vi "myRIOXGlobal.vi"() -> ()   [LabVIEW 2021]
uses:
  <vilib>/XNodeSupport/XNodeImage.ctl
  <vilib>/XNodeSupport/XNodeTerm4.ctl
  <vilib>/XNodeSupport/XNodeString.ctl
  <vilib>/XNodeSupport/XNodeVariant.ctl
  <vilib>/XNodeSupport/XNodeRect32.ctl
  <vilib>/XNodeSupport/XNodeInt.ctl
  <vilib>/XNodeSupport/XNodeBool.ctl
  <vilib>/XNodeSupport/XNodeTermDirection.ctl
  <vilib>/XNodeSupport/XNodeStandardHelpInfo.ctl
  <vilib>/XNodeSupport/XNodePath.ctl
  <vilib>/XNodeSupport/NI_XNodeSupport.lvlib
panel:
  out "AO Continuous Image":T1
  out "AO Continuous Help Info":T2={"Description"="Opens an FPGA reference to one or more analog output channels, which you use to perform continuous write operations. You must open a reference before you write values to an analog output channel.", "Path"=path "<helpdir>/elvis3vis.chm", "Tag"="elvis3vis_ao_continuous_sampling_open.html"}
  in  "AO Continuous Peripheral Name":string="AO (Continuous)"
  out "AI Continuous Image":T1
  out "AI Continuous Help Info":T2={"Description"="Opens an FPGA reference to one or more analog input channels, which you use to perform continuous read operations. You must open a reference before you read values from an analog input channel. ", "Path"=path "<helpdir>/elvis3vis.chm", "Tag"="myrioref_ai_continuous_sampling_open.html"}
  in  "AI Continuous Peripheral Name":string="AI (Continuous)"
  out "Max Range":T5={"Name"="Max Value", "Id"="Max Value", "Type"=variant(dbl[] []), "Bounds"={"Left"=16, "Top"=16, "Right"=24, "Bottom"=32}, "Input?"=TRUE, "Required?"=FALSE, "Recommended?"=TRUE, "Adaptive?"=FALSE, "Hidden?"=FALSE, "Direction"=enum."Auto", "Break Wire?"=FALSE, "English Name"=""}
  out "Min Range":T5={"Name"="Min Value", "Id"="Min Value", "Type"=variant(dbl[] []), "Bounds"={"Left"=8, "Top"=16, "Right"=16, "Bottom"=32}, "Input?"=TRUE, "Required?"=FALSE, "Recommended?"=TRUE, "Adaptive?"=FALSE, "Hidden?"=FALSE, "Direction"=enum."Auto", "Break Wire?"=FALSE, "English Name"=""}
  in  "Convert to SubVI OK Button":string="Convert"
  in  "Convert Fail Warning":string="Do you want to convert this VI to an empty VI? The current personality is incompatible with the peripheral. With an incompatible personality, you can only convert this VI to an empty VI."
  in  "Convert Success Warning":string="Do you want to convert this VI to a subVI? This operation disables error checking for FPGA personality at edit time."
  out "Timer IRQ Help Info":T2={"Description"="Creates timer interrupts.", "Path"=path "<helpdir>/myrioreference.chm", "Tag"="myrioref_create_timer_irq.html"}
  out "DI IRQ Help Info":T2={"Description"="Registers digital input interrupts.", "Path"=path "<helpdir>/myrioreference.chm", "Tag"="myrioref_register_di_irq.html"}
  out "AI IRQ Help Info":T2={"Description"="Registers analog input interrupts.", "Path"=path "<helpdir>/myrioreference.chm", "Tag"="myrioref_register_ai_irq.html"}
  in  "Timer IRQ Peripheral Name":string="Timer IRQ"
  in  "DI IRQ Peripheral Name":string="DI IRQ"
  in  "AI IRQ Peripheral Name":string="AI IRQ"
  out "Timer IRQ Image":T1
  out "DI IRQ Image":T1
  out "AI IRQ Image":T1
  out "DO Block Help Info":T2={"Description"="Opens a reference to one or more digital output channels, which you use to perform n samples write operations. You must open a reference before you write values to an digital output channel.", "Path"=path "<helpdir>/myrioreference.chm", "Tag"="myrioref_do_ns_open.html"}
  in  "DO Block Peripheral Name":string="DO (N Samples)"
  out "DO Block Image":T1
  out "DI Block Help Info":T2={"Description"="Opens a reference to one or more digital input channels, which you use to perform n samples write operations. You must open a reference before you read values from an digital input channel.", "Path"=path "<helpdir>/myrioreference.chm", "Tag"="myrioref_di_ns_open.html"}
  in  "DI Block Peripheral Name":string="DI (N Samples)"
  out "DI Block Image":T1
  out "AudioOut Block Help Info":T2={"Description"="Opens a reference to one or more audio output channels, which you use to perform n samples write operations. You must open a reference before you write values to an audio output channel.", "Path"=path "<helpdir>/myrioreference.chm", "Tag"="myrioref_audio_output_ns_open.html"}
  in  "AudioOut Block Peripheral Name":string="AudioOut (N Samples)"
  out "AudioOut Block Image":T1
  out "AudioIn Block Help Info":T2={"Description"="Opens a reference to one or more audio input channels, which you use to perform n samples read operations. You must open a reference before you read values from an audio input channel.", "Path"=path "<helpdir>/myrioreference.chm", "Tag"="myrioref_audio_input_ns_open.html"}
  in  "AudioIn Block Peripheral Name":string="AudioIn (N Samples)"
  out "AudioIn Block Image":T1
  out "AO Block Help Info":T2={"Description"="Opens a reference to one or more analog output channels, which you use to perform n samples write operations. You must open a reference before you write values to an analog output channel.", "Path"=path "<helpdir>/myrioreference.chm", "Tag"="myrioref_analog_output_ns_open.html"}
  in  "AO Block Peripheral Name":string="AO (N Samples)"
  out "AO Block Image":T1
  out "AI Block Help Info":T2={"Description"="Opens a reference to one or more analog input channels, which you use to perform n samples read operations. You must open a reference before you read values from an analog input channel.", "Path"=path "<helpdir>/myrioreference.chm", "Tag"="myrioref_analog_input_ns_open.html"}
  in  "AI Block Peripheral Name":string="AI (N Samples)"
  out "AI Block Image":T1
  out "SPI Help Info":T2={"Description"="Opens a reference to a serial peripheral interface (SPI) channel. You must open a reference before you use an SPI channel to write/read data to/from an SPI slave device.", "Path"=path "<helpdir>/myrioreference.chm", "Tag"="myrioref_spiopen.html"}
  out "PWM Help Info":T2={"Description"="Opens a reference to a pulse width modulation (PWM) channel. You must open a reference before you use a PWM channel to generate PWM signals.", "Path"=path "<helpdir>/myrioreference.chm", "Tag"="myrioref_pwmopen.html"}
  out "I2C Help Info":T2={"Description"="Opens a reference to an Inter-Integrated Circuit (I2C) channel. You must open a reference before you use an I2C channel to write/read data to/from an I2C slave device.", "Path"=path "<helpdir>/myrioreference.chm", "Tag"="myrioref_i2copen.html"}
  out "Encoder Help Info":T2={"Description"="Opens a reference to an encoder channel. You must open a reference before you use an encoder channel to read and decode signals from an encoder.", "Path"=path "<helpdir>/myrioreference.chm", "Tag"="myrioref_encoderopen.html"}
  out "DIO Help Info":T2={"Description"="Opens a reference to one or more digital I/O channels. You must open a reference before you read or write values.", "Path"=path "<helpdir>/myrioreference.chm", "Tag"="myrioref_dioopen.html"}
  out "AO Help Info":T2={"Description"="Opens a reference to one or more analog output channels. You must open a reference before you write values to an analog output channel.", "Path"=path "<helpdir>/myrioreference.chm", "Tag"="myrioref_aoopen.html"}
  out "AI Help Info":T2={"Description"="Opens a reference to one or more analog input channels. You must open a reference before you read values from an analog input channel.", "Path"=path "<helpdir>/myrioreference.chm", "Tag"="myrioref_aiopen.html"}
  out "Accelerometer Help Info":T2={"Description"="Opens a reference to one or more accelerometer channels. You must open a reference before you read values from an accelerometer channel.", "Path"=path "<helpdir>/myrioreference.chm", "Tag"="myrioref_accopen.html"}
  out "IP Address Term Constant":T5={"Name"="IP Address", "Id"="IP Address", "Type"=variant(string ""), "Bounds"={"Left"=0, "Top"=0, "Right"=8, "Bottom"=8}, "Input?"=TRUE, "Required?"=TRUE, "Recommended?"=FALSE, "Adaptive?"=FALSE, "Hidden?"=FALSE, "Direction"=enum."Auto", "Break Wire?"=FALSE, "English Name"=""}
  out "Allow Multiple Opens Term Constant":T5={"Name"="Allow multiple opens?", "Id"="Allow multiple opens?", "Type"=variant(bool FALSE), "Bounds"={"Left"=8, "Top"=0, "Right"=16, "Bottom"=16}, "Input?"=TRUE, "Required?"=FALSE, "Recommended?"=FALSE, "Adaptive?"=FALSE, "Hidden?"=FALSE, "Direction"=enum."Auto", "Break Wire?"=FALSE, "English Name"=""}
  out "Channel Names Term Constant":T5={"Name"="Channel Names", "Id"="Channel Names", "Type"=variant(tag[] []), "Bounds"={"Left"=0, "Top"=8, "Right"=8, "Bottom"=16}, "Input?"=TRUE, "Required?"=TRUE, "Recommended?"=FALSE, "Adaptive?"=FALSE, "Hidden?"=FALSE, "Direction"=enum."Auto", "Break Wire?"=FALSE, "English Name"=""}
  out "Channel Name Term Constant":T5={"Name"="Channel Name", "Id"="Channel Name", "Type"=variant(tag ""), "Bounds"={"Left"=0, "Top"=8, "Right"=8, "Bottom"=16}, "Input?"=TRUE, "Required?"=TRUE, "Recommended?"=FALSE, "Adaptive?"=FALSE, "Hidden?"=FALSE, "Direction"=enum."Auto", "Break Wire?"=FALSE, "English Name"=""}
  out "Error Out Term Constant":T5={"Name"="error out", "Id"="error out", "Type"=variant(errorcluster {"status"=FALSE, "code"=0, "source"=""}), "Bounds"={"Left"=24, "Top"=24, "Right"=32, "Bottom"=32}, "Input?"=FALSE, "Required?"=FALSE, "Recommended?"=TRUE, "Adaptive?"=FALSE, "Hidden?"=FALSE, "Direction"=enum."Auto", "Break Wire?"=FALSE, "English Name"=""}
  out "Error In Term Constant":T5={"Name"="error in (no error)", "Id"="error in (no error)", "Type"=variant(errorcluster {"status"=FALSE, "code"=0, "source"=""}), "Bounds"={"Left"=0, "Top"=24, "Right"=8, "Bottom"=32}, "Input?"=TRUE, "Required?"=FALSE, "Recommended?"=TRUE, "Adaptive?"=FALSE, "Hidden?"=FALSE, "Direction"=enum."Auto", "Break Wire?"=FALSE, "English Name"=""}
  in  "Error":string="The current personality or target does not support this VI."
  in  "Error Details":string="The current personality or target does not support this VI. Switch to another personality or change the current target."
  in  "SPI Peripheral Name":string="SPI"
  in  "PWM Peripheral Name":string="PWM"
  in  "I2C Peripheral Name":string="I2C"
  in  "Encoder Peripheral Name":string="Encoder"
  in  "AO Peripheral Name":string="AO"
  in  "DIO Peripheral Name":string="DIO"
  out "SPI Image":T1
  out "PWM Image":T1
  out "I2C Image":T1
  in  "Accelerometer Peripheral Name":string="Accelerometer"
  out "Accelerometer Image":T1
  in  "AI Peripheral Name":string="AI"
  out "Encoder Image":T1
  out "DIO Image":T1
  out "AO Image":T1
  out "AI Image":T1
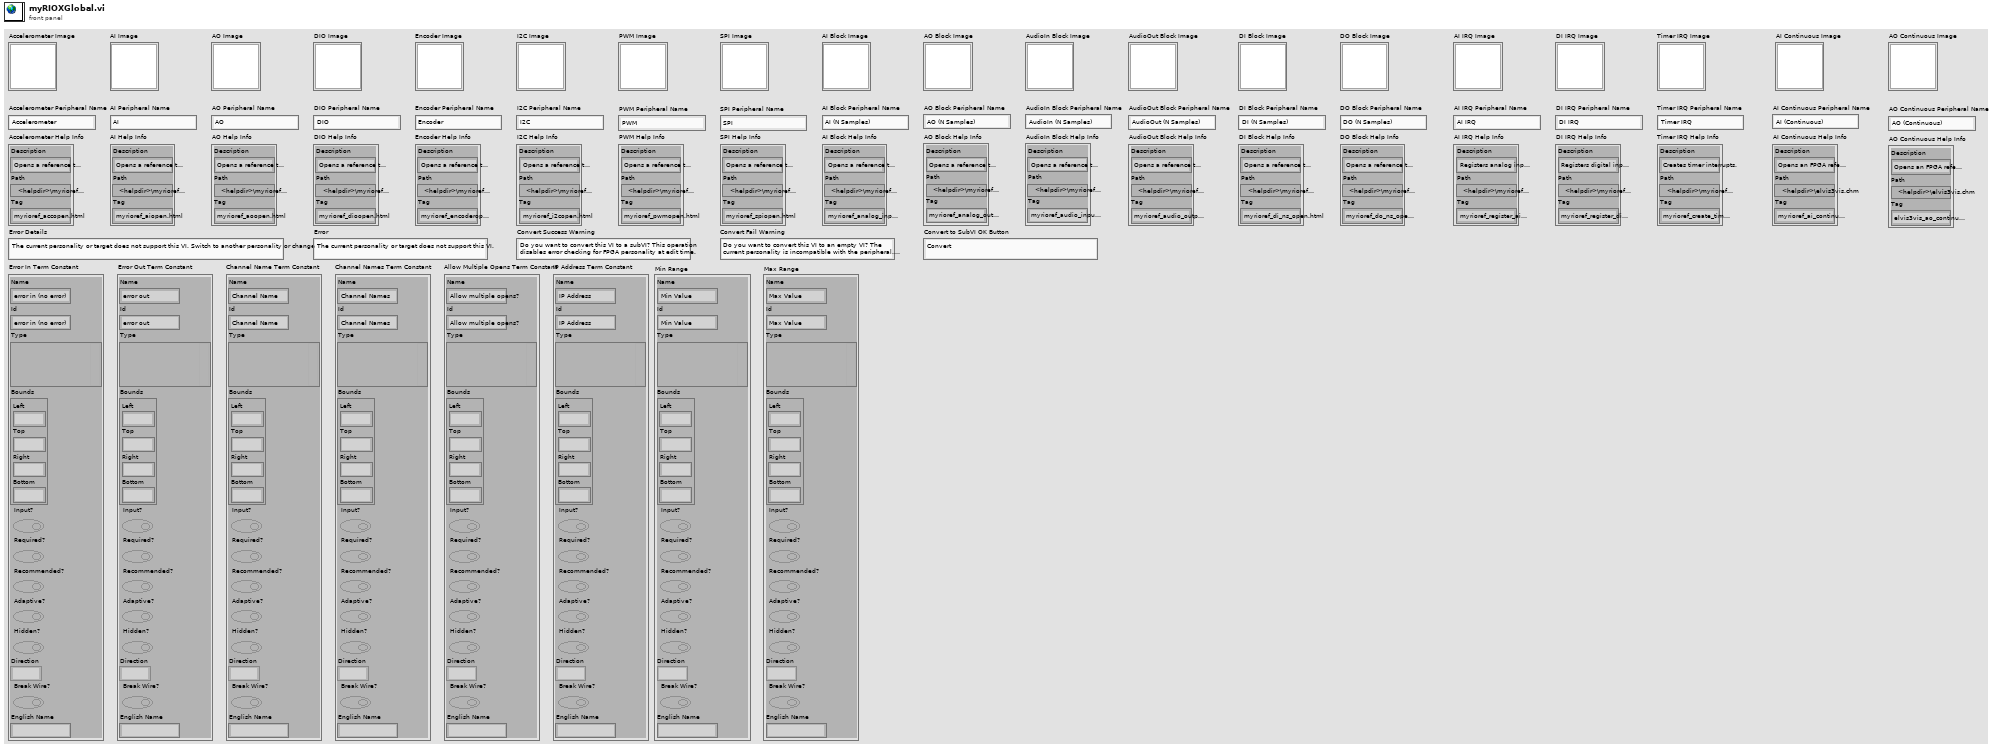
[diagram p1: front panel]
types:
  T1 = typedef "NI_XNodeSupport.lvlib/XNodeImage.ctl" = picture
  T2 = typedef "NI_XNodeSupport.lvlib/XNodeStandardHelpInfo.ctl" = cluster{"Description":T3, "Path":T4, "Tag":T3}
  T3 = typedef "NI_XNodeSupport.lvlib/XNodeString.ctl" = string
  T4 = typedef "NI_XNodeSupport.lvlib/XNodePath.ctl" = path
  T5 = typedef "NI_XNodeSupport.lvlib/XNodeTerm4.ctl" = cluster{"Name":T3, "Id":T3, "Type":T6, "Bounds":T7, "Input?":T9, "Required?":T9, "Recommended?":T9, "Adaptive?":T9, "Hidden?":T9, "Direction":T10, "Break Wire?":T9, "English Name":T3}
  T6 = typedef "NI_XNodeSupport.lvlib/XNodeVariant.ctl" = variant
  T7 = typedef "NI_XNodeSupport.lvlib/XNodeRect32.ctl" = cluster{"Left":T8, "Top":T8, "Right":T8, "Bottom":T8}
  T8 = typedef "NI_XNodeSupport.lvlib/XNodeInt.ctl" = i32
  T9 = typedef "NI_XNodeSupport.lvlib/XNodeBool.ctl" = bool
  T10 = typedef "NI_XNodeSupport.lvlib/XNodeTermDirection.ctl" = enum32{"Auto", "Up", "Down", "Left", "Right", "Center"}
diagram:
